vi "Keithley 2002 Single Read.vi"(0 "GPIB address":string="16", 1 "source (imm:1)":u16(ring)=1 items=["hold", "immediate", "timer", "manual", "bus", "trigger link", "external"], 2 "timer value (secs)":dbl=0.001 min=0.001 max=999999.999 format="%.3f", 3 "error in":T1) -> (4 "units":string, 5 "reading #":dbl, 6 "measurement":dbl format="%.6e", 8 "channel #":dbl, 9 "error out":T1)   [LabVIEW 2020]
doc: "This VI is used to configure the Measure Layer (Trigger) and take a single measurement. The buffer is not used for this reading. The instrument simply returns the last measurement taken.\n\nTo configure the function to read use one of the Config VI's. For example, to configure DC volts, use the VDC Config VI."
panel:
  out "time and date stamp":string
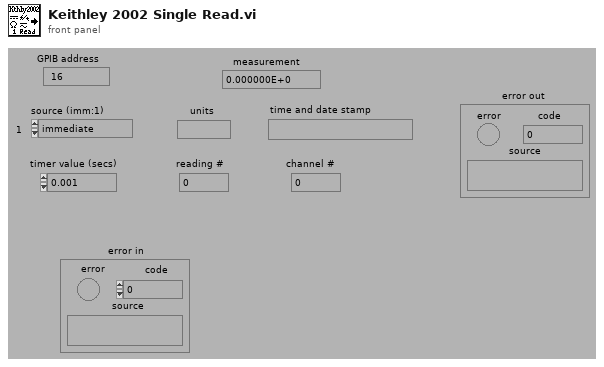
[diagram p1: front panel]
types:
  T1 = cluster{"error":bool, "code":i32, "source":string}
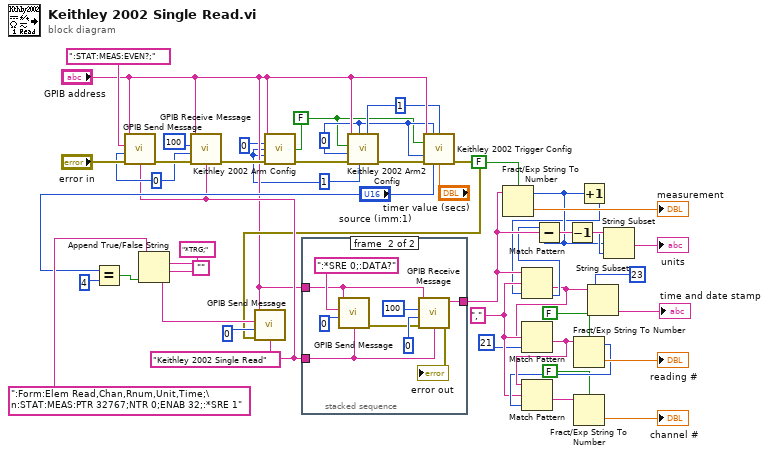
[diagram p0: block diagram]
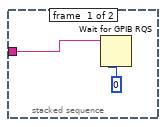
[diagram p2: hidden frame]
diagram:
  w9 = ","
  w35 = 0
  w16 = 1
  w15 = 0
  w13 = FALSE
  w11 = 1
  w33 = "Keithley 2002 Single Read"
  n1 = Equal?(x="source (imm:1)", y=4) -> (x = y?=w44:bool)
  n2 = call "GPIB Send Message.vi"("address string"="GPIB address", "write buffer"=":STAT:MEAS:EVEN?;", "source"=w33, "write mode (set END:0)"=w35, "error in"="error in") -> ("error out"=w39:T1)  [unwired: 2 in, 2 out]
  n3 = Append True/False String(1:w44, 2:"", 3:"*TRG;", 4:":Form:Elem Read,Chan,Rnum,Unit,Time;\n:STAT:MEAS:PTR 32767;NTR 0;ENAB 32;:*SRE 1") -> (0:w41:string)
  n4 = call "GPIB Receive Message.vi"("address string"="GPIB address", "byte count"=100, "source"=w33, "read mode"=w35, "error in"=w39) -> ("error out"=w21:T1)  [unwired: 2 in, 2 out]
  n5 = call "Keithley 2002 Arm Config.vi"("GPIB address"="GPIB address", "count (set:0)"=0, "count value"=w11, "direction"=w13, "source (imm:1)"=w11, "error in"=w21) -> ("error out"=w20:T1)  [unwired: 9 in]
  n6 = stacked-sequence {
    tunnel: "GPIB address" -> [w47 w50]
    tunnel: w33 -> [_ w51]
    tunnel: [_ w49] -> w28
    frame #0 {
      n7 = Wait for GPIB RQS(3:0, 4:w47) -> ()  [unwired: 1 in, 2 out]
    }
    frame #1 {
      n8 = call "GPIB Send Message.vi"("address string"=w50, "write buffer"=":*SRE 0;:DATA?", "source"=w51, "write mode (set END:0)"=0) -> ("error out"=w53:T1)  [unwired: 3 in, 2 out]
      n9 = call "GPIB Receive Message.vi"("address string"=w50, "byte count"=100, "source"=w51, "read mode"=0, "error in"=w53) -> ("read buffer"=w49:string, "error out"=→"error out":T1)  [unwired: 2 in, 1 out]
    }
  }
  n10 = call "Keithley 2002 Arm2 Config.vi"("count value"=w16, "source (imm:1)"=w11, "count (set:0)"=w15, "error in"=w20, "delay (secs)"=w15, "direction"=w13, "GPIB address"="GPIB address") -> ("error out"=w19:T1)  [unwired: 4 in]
  n11 = call "Keithley 2002 Trigger Config.vi"("GPIB address"="GPIB address", "count (set:0)"=w15, "count value"=w16, "direction"=w13, "delay (secs)"=w15, "error in"=w19, "source (imm:1)"="source (imm:1)", "timer value (secs)"="timer value (secs)") -> ("error out"=w18:T1)  [unwired: 7 in]
  n12 = call "GPIB Send Message.vi"("address string"="GPIB address", "write buffer"=w41, "source"=w33, "write mode (set END:0)"=0, "error in"=w18) -> ()  [unwired: 2 in, 3 out]
  n13 = Fract/Exp String To Number(use system decimal point (T)=FALSE, string=w28) -> (offset past number=w10:i32, number=→"measurement":dbl)  [unwired: 2 in]
  n14 = Increment(x=w10) -> (x+1=w8:i32)
  n15 = Match Pattern(string=w28, regular expression=w9, offset (0)=w8) -> (after substring=w6:string, offset past match=w24:i32)  [unwired: 2 out]
  n16 = Match Pattern(string=w6, regular expression=w9, offset (0)=21) -> (after substring=w26:string)  [unwired: 3 out]
  n17 = Subtract(x=w24, y=w10) -> (x-y=w22:i32)
  n18 = Decrement(x=w22) -> (x-1=w23:i32)
  n19 = Fract/Exp String To Number(use system decimal point (T)=FALSE, string=w26) -> (offset past number=w25:i32, number=→"reading #":dbl)  [unwired: 2 in]
  n20 = Match Pattern(string=w26, regular expression=w9, offset (0)=w25) -> (after substring=w27:string)  [unwired: 3 out]
  n21 = Fract/Exp String To Number(use system decimal point (T)=FALSE, string=w27) -> (number=→"channel #":dbl)  [unwired: 2 in, 1 out]
  n22 = String Subset(string=w6, length (rest)=23) -> (substring=→"time and date stamp":string)  [unwired: 1 in]
  n23 = String Subset(string=w28, offset (0)=w10, length (rest)=w23) -> (substring=→"units":string)
